vi "Open Device.vi"   [LabVIEW 2019, in "D2XX-lv.lvlib"]
uses:
  D2XX-lv.lvlib
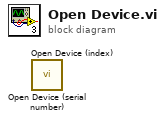
[diagram p0: block diagram]
diagram:
  n1 = call "Open Device (serial number).vi"() -> ()  [unwired: 10 in, 2 out]
  n2 = call "Open Device (index).vi"() -> ()  [unwired: 10 in, 2 out]
